vi "IO@WaitPortOff__Parameter.vi"(1 "ParamterIn":string) -> (0 "ParamterOut":string)   [LabVIEW 2019]
panel:
  in  "Message":string(combo)
  in  "TimeOut":string(combo)
  in  "PortSelect":string(combo)
  in  "Confirm":bool
  # "IO@WaitPortOn/Off $IOName(,$Timeout=XX,[[$label]]$Message)"
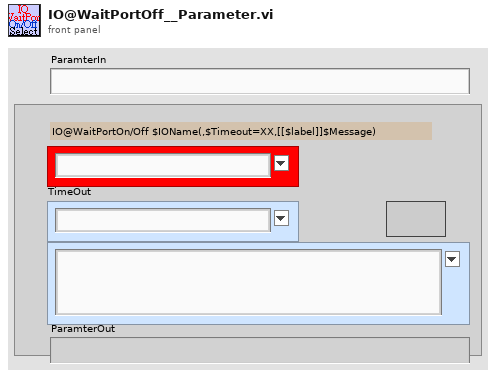
[diagram p1: front panel]
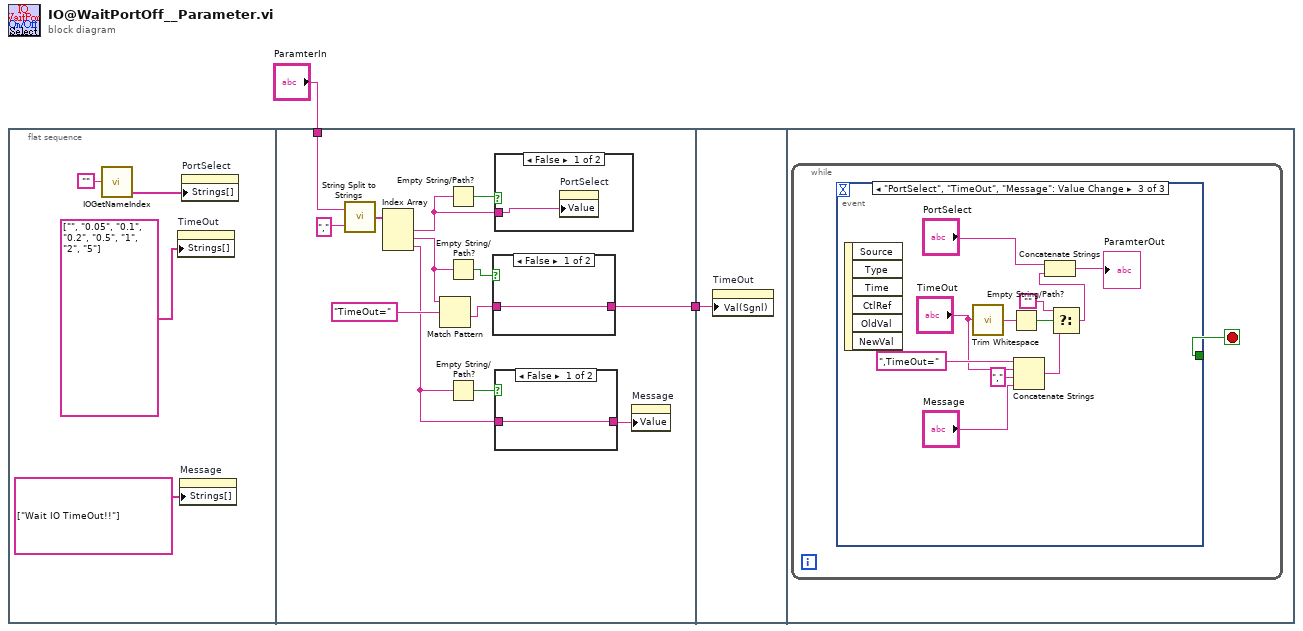
[diagram p0: block diagram]
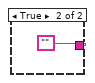
[diagram p2: hidden frame]
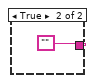
[diagram p3: hidden frame]
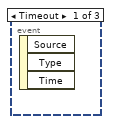
[diagram p5: hidden frame]
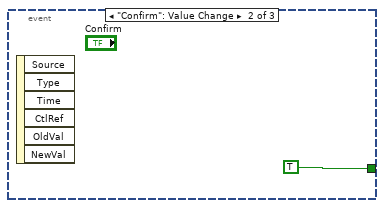
[diagram p6: hidden frame]
diagram:
  n1 = flat-sequence {
    tunnel: "ParamterIn" -> [w17]
    tunnel: [w7] -> w1
    tunnel: w1 -> [w25]
    frame #0 {
      n2 = call "IOGetNameIndex.vi"("PortName"="") -> ("PortNameList Out"=w5:string[])  [unwired: 3 in, 1 out]
      n3 = property on="TimeOut" class="CmbBox"("Strings[]"=string[] ["", "0.05", "0.1", "0.2", "0.5", "1", "2", "5"] ("Strings []")) -> ()  [unwired: 2 in, 2 out]
      n4 = property on="Message" class="CmbBox"("Strings[]"=string[] ["Wait IO TimeOut!!"] ("Strings []")) -> ()  [unwired: 2 in, 2 out]
      n5 = property on="PortSelect" class="CmbBox"("Strings[]"=w5) -> ()  [unwired: 2 in, 2 out]
    }
    frame #1 {
      n6 = call "String Split to Strings.vi"("search string/char (-)"=",", "String"=w17) -> ("Array"=w19:string[])
      n7 = Index Array(array=w19) -> (element #1=w15:string, element #2=w13:string, element #3=w9:string)  [unwired: 3 in]
      n8 = Match Pattern(string=w13, regular expression="TimeOut=") -> (after substring=w12:string)  [unwired: 1 in, 3 out]
      n9 = Empty String/Path?(string/path=w15) -> (empty?=w16:bool)
      n10 = Empty String/Path?(string/path=w13) -> (empty?=w14:bool)
      n11 = Empty String/Path?(string/path=w9) -> (empty?=w10:bool)
      n12 = case shown="False" w14 {
        tunnel: [w22 ""] -> w7
        tunnel: w12 -> [w22 _]
        frame False {
        }
        frame True {
        }
      }
      n13 = case shown="False" w16 {
        tunnel: w15 -> [w24 _]
        frame False {
          n14 = property on="PortSelect" class="CmbBox"("Value"=w24) -> ()  [unwired: 2 in, 2 out]
        }
        frame True {
        }
      }
      n15 = case shown="False" w10 {
        tunnel: [w20 ""] -> w8
        tunnel: w9 -> [w20 _]
        frame False {
        }
        frame True {
        }
      }
      n16 = property on="Message" class="CmbBox"("Value"=w8) -> ()  [unwired: 2 in, 2 out]
    }
    frame #2 {
      n17 = property on="TimeOut" class="CmbBox"("Val(Sgnl)"=w25) -> ()  [unwired: 2 in, 2 out]
    }
    frame #3 {
      n18 = while {
        stop <- w26 stop-if-true
        n19 = event shown="[2] \"PortSelect\", \"TimeOut\", \"Message\": Value Change" {
          selector: _ -> [_ _ _]
          dyn-events: _ -> [_ _ _]
          timeout: _ -> [_ _ _]
          tunnel: [_ TRUE _] -> w26
          event Timeout {
            n20 = event-data() -> ()  [unwired: 1 in, 3 out]
          }
          event "Confirm": Value Change {
            n21 = event-data() -> ()  [unwired: 1 in, 6 out]
          }
          event "PortSelect", "TimeOut", "Message": Value Change {
            n22 = event-data() -> ()  [unwired: 1 in, 6 out]
            n23 = call <vilib>:"Trim Whitespace.vi"("string"="TimeOut") -> ("trimmed string"=w32:string)  [unwired: 1 in]
            n24 = Empty String/Path?(string/path=w32) -> (empty?=w33:bool)
            n25 = Concatenate Strings(",TimeOut=" ("string"), "TimeOut", "," ("string"), "Message") -> (w35:string)
            n26 = Select(t="", s=w33, f=w35) -> (s? t:f=w30:string)
            n27 = Concatenate Strings("PortSelect", w30) -> (→"ParamterOut":string)
          }
        }
      }
    }
  }
